vi "New Ball Stack.vi"(4 "Top Stack Speed":dbl=0.5, 5 "BottomMS":bool, 6 "TopMS":bool, 7 "CupMS":bool, 8 "spinOut?":bool, 9 "Suck?":bool) -> (0 "Floor":dbl, 1 "Middle":dbl, 2 "Top":dbl)   [LabVIEW 2011]
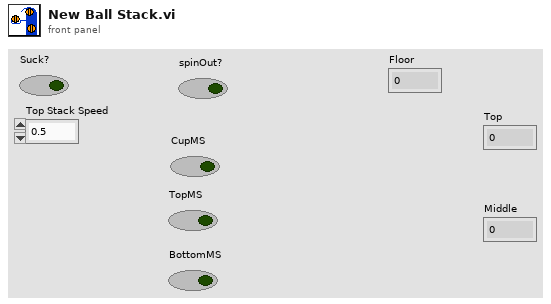
[diagram p1: front panel]
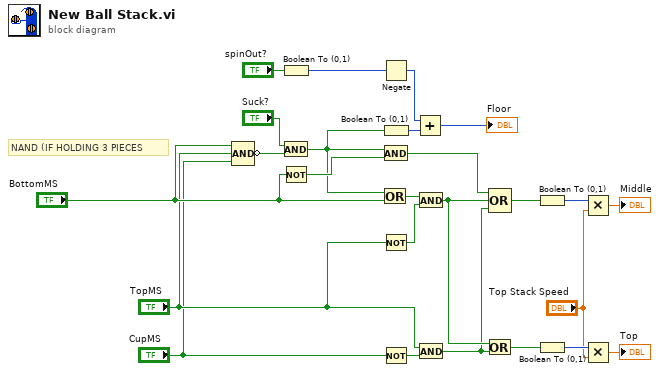
[diagram p0: block diagram]
diagram:
  # "NAND (IF HOLDING 3 PIECES"
  n1 = Compound Arithmetic op=AND("BottomMS", "TopMS", "CupMS") -> (invert w3:bool)
  n2 = Boolean To (0,1)(Boolean="spinOut?") -> (0, 1=w24:i16)
  n3 = And(x="Suck?", y=w3) -> (x .and. y?=w2:bool)
  n4 = Not(x="BottomMS") -> (.not. x?=w14:bool)
  n5 = Or(x=w2, y="BottomMS") -> (x .or. y?=w20:bool)
  n6 = Negate(x=w24) -> (-x=w23:i16)
  n7 = Boolean To (0,1)(Boolean=w2) -> (0, 1=w22:i16)
  n8 = And(x=w2, y=w14) -> (x .and. y?=w13:bool)
  n9 = Not(x="TopMS") -> (.not. x?=w19:bool)
  n10 = Not(x="CupMS") -> (.not. x?=w18:bool)
  n11 = Add(x=w23, y=w22) -> (x+y=→"Floor":i16)
  n12 = And(x=w20, y=w19) -> (x .and. y?=w12:bool)
  n13 = And(x="TopMS", y=w18) -> (x .and. y?=w11:bool)
  n14 = Or(x=w12, y=w11) -> (x .or. y?=w17:bool)
  n15 = Compound Arithmetic op=OR(w13, w12, w11) -> (w8:bool)
  n16 = Boolean To (0,1)(Boolean=w8) -> (0, 1=w10:i16)
  n17 = Boolean To (0,1)(Boolean=w17) -> (0, 1=w16:i16)
  n18 = Multiply(x=w10, y="Top Stack Speed") -> (x*y=→"Middle":dbl)
  n19 = Multiply(x=w16, y="Top Stack Speed") -> (x*y=→"Top":dbl)
